vi "Get Plot Visibility (WFChart).vi"(8 "error in (no error)":errorcluster, 11 "WaveformChart in":refnum<vi>) -> (0 "error out":errorcluster, 2 "Plot.Visible":bool[](array[boolean]))   [LabVIEW 2019, in "Instrument.Lockin.lvlib" / "Instrument UI.Lockin.lvclass"]
uses:
  Instrument UI.Lockin.lvclass
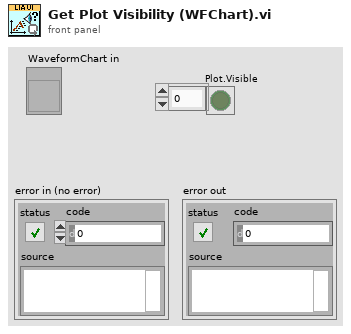
[diagram p1: front panel]
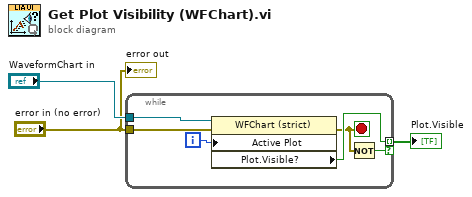
[diagram p0: block diagram]
diagram:
  n1 = while {
    tunnel: [w7] -> w3 mode=indexing if=w6
    tunnel: "WaveformChart in" -> [w9]
    tunnel: "error in (no error)" -> [w8]
    i -> [w4]
    stop <- w5 stop-if-true
    n2 = property on="Property Node" class="WFChart (strict)"(reference=w9, error in=w8, "Active Plot"=w4) -> (error out=w5:errorcluster, "Plot.Visible?"=w7:bool)  [unwired: 1 out]
    n3 = Not(x=w5) -> (.not. x?=w6:bool)
  }
  "Plot.Visible" <- w3
  "error out" <- "error in (no error)"
